vi "ma_Check Limit X, x0, dx.vi"(0 "X":dbl[](array[numeric]) format="%0.2f", 1 "x0":dbl format="%0.2f", 2 "dx":dbl format="%0.2f", 3 "error in":errorcluster) -> (8 "limit spec ok":bool, 10 "error out":errorcluster)   [LabVIEW 2020, in "NI_MAPro.lvlib"]
uses:
  NI_MAPro.lvlib
  NI_MABase.lvlib
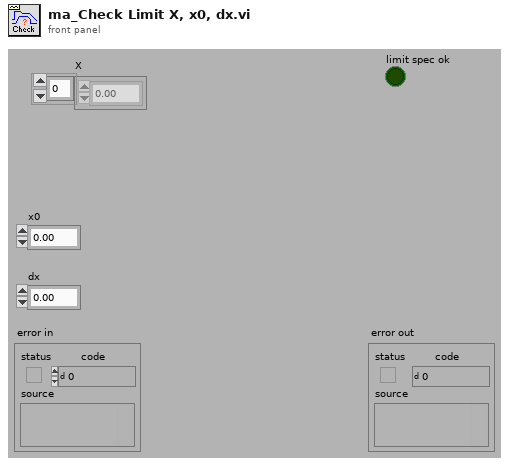
[diagram p1: front panel]
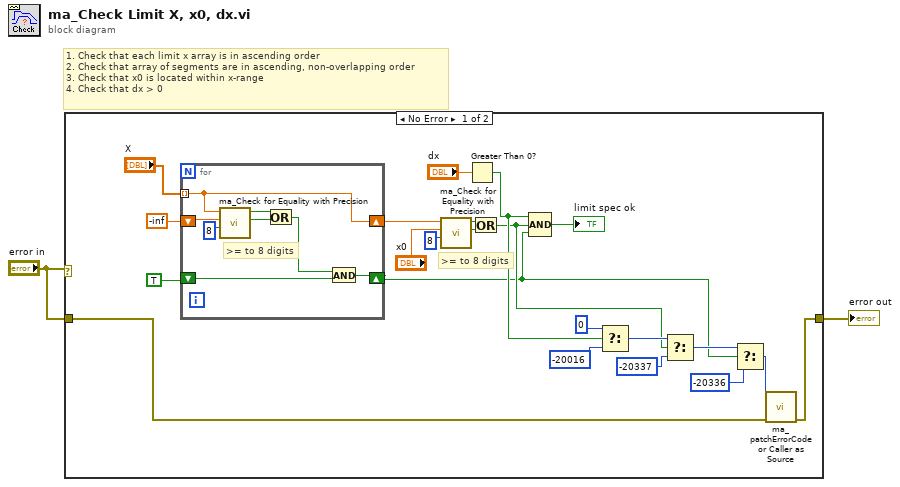
[diagram p0: block diagram]
diagram:
  # "1. Check that each limit x array is in ascending order\n2. Check that array of segments are in ascending, non-overlapping order\n3. Check that x0 is located within x-range\n4. Check that dx > 0"
  n1 = case shown="No Error" "error in" {
    tunnel: [w21 w33] -> w1
    tunnel: "error in" -> [w22 w33]
    frame No Error {
      # ">= to 8 digits"
      n2 = for {
        shift-right: [w25] -> w8
        shift-left: -inf -> [w30]
        tunnel: "X" -> [w25] mode=indexing
        shift-right: [w31] -> w3
        shift-left: TRUE -> [w32]
        # ">= to 8 digits"
        n3 = call "ma_Check for Equality with Precision.vi"("precision"=8, "n2"=w30, "n1"=w25) -> ("n1 > n2?"=w28:bool, "equal (within precision)"=w29:bool)  [unwired: 7 out]
        n4 = Or(x=w29, y=w28) -> (x .or. y?=w27:bool)
        n5 = And(x=w27, y=w32) -> (x .and. y?=w31:bool)
      }
      n6 = call "ma_Check for Equality with Precision.vi"("precision"=8, "n2"="x0", "n1"=w8) -> ("n1 > n2?"=w6:bool, "equal (within precision)"=w7:bool)  [unwired: 7 out]
      n7 = Greater Than 0?(x="dx") -> (x > 0?=w12:bool)
      n8 = Or(x=w7, y=w6) -> (x .or. y?=w5:bool)
      n9 = Compound Arithmetic op=AND(w12, w5, w3) -> (→"limit spec ok":bool)
      n10 = Select(t=0 ("Error Code"), s=w12, f=-20016) -> (s? t:f=w13:i32)
      n11 = Select(t=w13, s=w5, f=-20337 ("Error Code")) -> (s? t:f=w17:i32)
      n12 = Select(t=w17, s=w3, f=-20336 ("Error Code")) -> (s? t:f=w11:i32)
      n13 = call "ma_patchErrorCode or Caller as Source.vi"("error in (no error)"=w22, "error code"=w11) -> ("error out"=w21:errorcluster)  [unwired: 2 in, 7 out]
    }
    frame Error {
    }
  }
  "error out" <- w1
